vi "Get File Info.vi"(8 "error in (no error)":errorcluster, 11 "midi file in":refnum<class "midi file.lvclass">) -> (0 "error out":errorcluster, 2 "File Info":T1, 3 "midi file out":refnum<class "midi file.lvclass">)   [LabVIEW 2020, in "MIDIllan.lvlib" / "midi file.lvclass"]
uses:
  midi file.lvclass
  file info.ctl
  midi file.lvclass/midi file.ctl
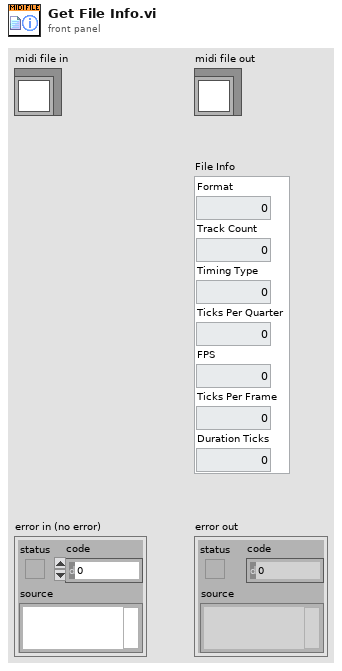
[diagram p1: front panel]
types:
  T1 = typedef "MIDIllan.lvlib/midi file.lvclass/file info.ctl" = cluster{"Format":i32, "Track Count":i32, "Timing Type":i32, "Ticks Per Quarter":i32, "FPS":sgl, "Ticks Per Frame":i32, "Duration Ticks":u32}
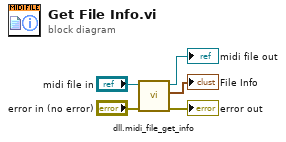
[diagram p0: block diagram]
diagram:
  n1 = call "dll.midi_file_get_info.vi"("error in (no error)"="error in (no error)", "midi file in"="midi file in") -> ("error out"=→"error out":errorcluster, "File Info Cluster"=→"File Info":T1, "midi file out"=→"midi file out":refnum<class "midi file.lvclass">)  [unwired: 7 in]
